vi "OpenErrorLog.vi"(5 "Error In":errorcluster) -> (19 "Error Out":errorcluster)   [LabVIEW 2019, in "Error handler.lvclass"]
uses:
  Error handler.lvclass
  ErrorLogFile_class/ErrorLogFile.lvclass
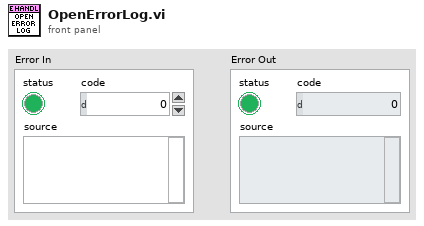
[diagram p1: front panel]
types:
  T1 = typedef "Error handler.lvclass/ObjectAttributes.ctl" = cluster{"ErrorBroadcastEvent":refnum<user-event>, "LoadFPOnError":bool, "ErrorLogFile":refnum<class "ErrorLogFile.lvclass">, "Testing":bool, "Name":string}
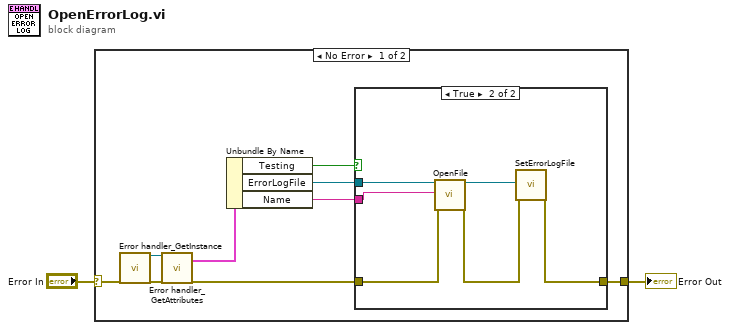
[diagram p0: block diagram]
diagram:
  n1 = case shown="No Error" "Error In" {
    selector: "Error In" -> [w9 w19]
    tunnel: [w5 w19] -> w1
    frame No Error {
      n2 = call "Error handler_GetInstance.vi"("error in"=w9) -> ("reference out"=w10:refnum<class "Error handler.lvclass">, "error out"=w8:errorcluster)  [unwired: 14 in, 3 out]
      n3 = call "Error handler_GetAttributes.vi"("reference in"=w10, "error in (no error)"=w8) -> ("Data"=w11:T1, "error out"=w6:errorcluster)  [unwired: 14 in, 2 out]
      n4 = Unbundle By Name(w11) -> ("Testing"=w4:bool, "ErrorLogFile"=w7:refnum<class "ErrorLogFile.lvclass">, "Name"=w3:string)
      n5 = case shown="True" w4 {
        tunnel: w7 -> [_ w18]
        tunnel: w6 -> [w12 w17]
        tunnel: [w12 w14] -> w5
        tunnel: w3 -> [_ w13]
        frame False {
        }
        frame True {
          n6 = call-dynamic "OpenFile.vi"("object in"=w18, "Name"=w13, "Error In"=w17) -> ("object out"=w16:refnum<class "ErrorLogFile.lvclass">, "Error Out"=w15:errorcluster)  [unwired: 15 in]
          n7 = call "SetErrorLogFile.vi"("ErrorLogFile"=w16, "Error In"=w15) -> ("Error Out"=w14:errorcluster)  [unwired: 17 in]
        }
      }
    }
    frame Error {
    }
  }
  "Error Out" <- w1
